vi "Open Instrument.vi"(8 "error in (no error)":errorcluster, 11 "Instrument.VoltageSource in":refnum<class "Instrument.VoltageSource.lvclass">) -> (0 "error out":errorcluster, 3 "Instrument.VoltageSource out":refnum<class "Instrument.VoltageSource.lvclass">)   [LabVIEW 2016, in "Instrument.VoltageSource.lvclass"]
uses:
  Instrument.VoltageSource.lvclass
  Instrument.VoltageSource.lvclass/Instrument.VoltageSource.ctl
  <vilib>/DAQmx/create/channels.llb/DAQmx Create Channel (AO-Voltage-Basic).vi
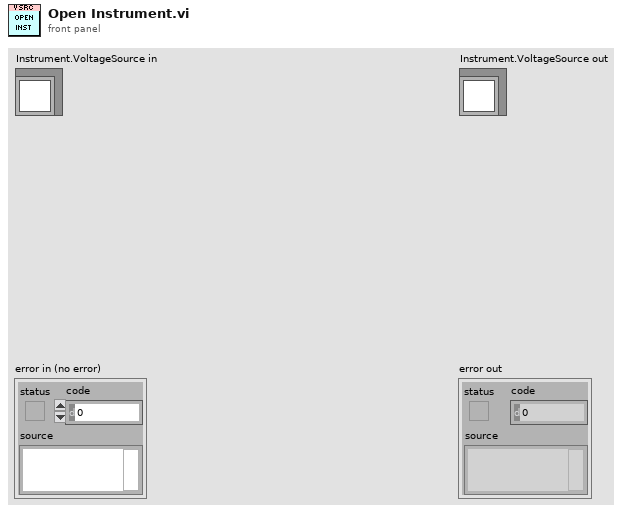
[diagram p1: front panel]
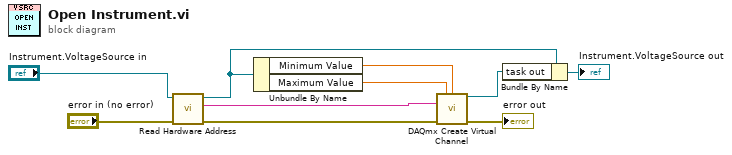
[diagram p0: block diagram]
diagram:
  n1 = call-dynamic "Read Hardware Address.vi"("error in (no error)"="error in (no error)", "Instrument in"="Instrument.VoltageSource in") -> ("error out"=w8:errorcluster, "Hardware Address"=w9:string, "Instrument out"=w1:refnum<class "Instrument.VoltageSource.lvclass">)  [unwired: 7 in]
  n2 = Unbundle By Name(w1) -> ("Minimum Value"=w5:dbl, "Maximum Value"=w4:dbl)
  n3 = call-poly <vilib>:"DAQmx Create Virtual Channel.vi"("maximum value"=w4, "minimum value"=w5, "physical channels"=w9, "error in"=w8) -> ("task out"=w3:refnum<k21>, "error out"=→"error out":errorcluster)  [unwired: 10 in]
  n4 = Bundle By Name(cluster=w1, "task out"=w3) -> (→"Instrument.VoltageSource out":refnum<class "Instrument.VoltageSource.lvclass">)
